vi "Calibrate VSEC.vi"(8 "error in (no error)":errorcluster, 9 "Position in":u32, 10 "Cree Comms in":refnum<class "Cree Communications.lvclass">, 11 "Calibration in":refnum<class "Calibration.lvclass">) -> (0 "error out":errorcluster, 1 "Position out":u32, 2 "Cree Comms out":refnum<class "Cree Communications.lvclass">, 3 "Calibration out":refnum<class "Calibration.lvclass">, 4 "Passed":bool, 6 "Fail Code":string)   [LabVIEW 2015, in "Calibration.lvclass"]
uses:
  Calibration.lvclass
  Classes/Cree Communications/Class/Cree Communications.lvclass
  Classes/Application/Class/Application.lvclass
  Test Class/Test Class.lvclass
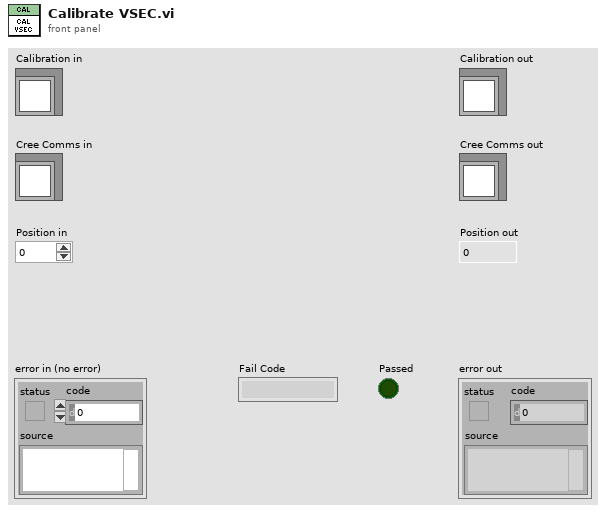
[diagram p1: front panel]
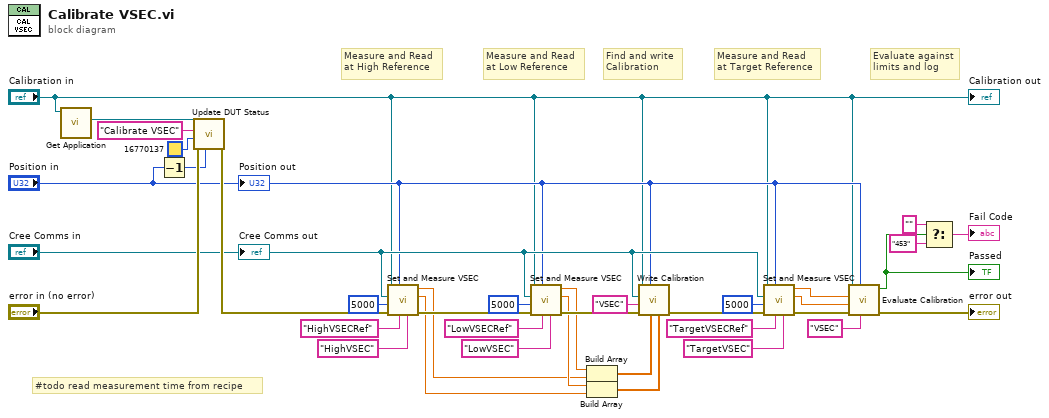
[diagram p0: block diagram]
diagram:
  # "#todo read measurement time from recipe"
  # "Evaluate against\nlimits and log"
  # "Measure and Read\nat Target Reference"
  # "Find and write\nCalibration"
  # "Measure and Read\nat Low Reference"
  # "Measure and Read\nat High Reference"
  n1 = call "Get Application.vi"("Test Class in"="Calibration in") -> ("Application.lvlib:Application.lvclass"=w1:refnum<class "Application.lvclass">)  [unwired: 9 in, 1 out]
  n2 = Decrement(x="Position in") -> (x-1=w6:u32)
  n3 = call "Update DUT Status.vi"("Position"=w6, "error in (no error)"="error in (no error)", "BG Color"=u32 16770137, "Message ('')"="Calibrate VSEC", "Application in"=w1) -> ("error out"=w36:errorcluster)  [unwired: 5 in, 1 out]
  n4 = call "Set and Measure VSEC.vi"("Header"="HighVSEC" ("Name"), "Name"="HighVSECRef", "Position in"="Position in", "error in (no error)"=w36, "Measurement Wait Time"=u32 5000, "Cree Comms in"="Cree Comms in", "Calibration in"="Calibration in") -> ("error out"=w30:errorcluster, "DSpic Measurement"=w27:dbl, "Actual Measurement"=w19:dbl)  [unwired: 2 in]
  n5 = call "Set and Measure VSEC.vi"("Header"="LowVSEC" ("Name"), "Name"="LowVSECRef", "Position in"="Position in", "error in (no error)"=w30, "Measurement Wait Time"=u32 5000, "Cree Comms in"="Cree Comms in", "Calibration in"="Calibration in") -> ("error out"=w29:errorcluster, "DSpic Measurement"=w26:dbl, "Actual Measurement"=w28:dbl)  [unwired: 2 in]
  n6 = Build Array(w28, w19) -> (w24:dbl[])
  n7 = Build Array(w26, w27) -> (w25:dbl[])
  n8 = call "Write Calibration.vi"("DSPic Measurements"=w25, "Actual Measurements"=w24, "Position in"="Position in", "error in (no error)"=w29, "Calibration Type"="VSEC", "Cree Comms in"="Cree Comms in", "Calibration in"="Calibration in") -> ("error out"=w22:errorcluster)  [unwired: 4 in]
  n9 = call "Set and Measure VSEC.vi"("Header"="TargetVSEC" ("Name"), "Name"="TargetVSECRef", "Position in"="Position in", "error in (no error)"=w22, "Measurement Wait Time"=u32 5000, "Cree Comms in"="Cree Comms in", "Calibration in"="Calibration in") -> ("error out"=w15:errorcluster, "DSpic Measurement"=w11:dbl, "Actual Measurement"=w12:dbl)  [unwired: 2 in]
  n10 = call "Evaluate Calibration.vi"("Calibration Type"="VSEC" ("Name"), "Position"="Position in", "Error in"=w15, "DSPic Measurement"=w11, "Actual Measurement"=w12, "Calibration in"="Calibration in") -> ("Error out"=→"error out":errorcluster, "Passed"=w9:bool)  [unwired: 4 in]
  "Passed" <- w9
  n11 = Select(t="", s=w9, f="453") -> (s? t:f=→"Fail Code":string)
  "Calibration out" <- "Calibration in"
  "Position out" <- "Position in"
  "Cree Comms out" <- "Cree Comms in"
